vi "Start Process.vi"(8 "error in":errorcluster) -> (0 "error out":errorcluster)   [LabVIEW 2015]
uses:
  Message Queue/Message Queue.lvlib
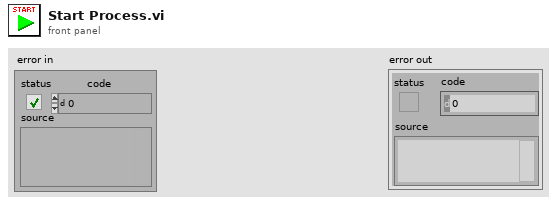
[diagram p1: front panel]
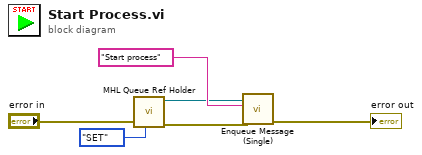
[diagram p0: block diagram]
diagram:
  n1 = call "MHL Queue Ref Holder.vi"("Action"=enum16{"GET", "SET"}."SET", "error in"="error in") -> ("error out"=w2:errorcluster, "Input Message Queue"=w3:refnum<queue>)  [unwired: 8 in]
  n2 = call "Enqueue Message (Single).vi"("error in (no error)"=w2, "Message"="Start process", "Message Queue"=w3) -> ("error out"=→"error out":errorcluster)  [unwired: 7 in, 1 out]
